vi "Servo Set Pulse Width N Channels.vi"(8 "Error In":errorcluster, 9 "Pulse Widths (uS)":u16[](array[numeric]), 10 "Servo Channels":u8[](array[numeric]), 11 "LINX Resource":T1) -> (0 "Error Out":errorcluster, 3 "LINX Resource":T1)   [LabVIEW 2014, in "LMH-LINX.lvlib" / "Servo.lvlib"]
doc: "Set the pulse width of the specified servo channel.\n\nA pulse width of 1500uS is typically the center point of rotation (90 degrees). Most servos can rotate between 1000 and 2000 uS but the actual limits will vary depending on the specific servo.s"
uses:
  <vilib>/MakerHub/LINX/Public/Sensors/Motion/Servo/Servo.lvlib
  <vilib>/MakerHub/LINX/Private/Type Defs/LINX Ref.ctl
  <vilib>/MakerHub/LINX/Private/Type Defs/Platform.ctl
  <vilib>/MakerHub/LINX/Private/Type Defs/Interface.ctl
  <vilib>/MakerHub/LINX/Private/Device/Type Defs/LINX Device Config.ctl
  <vilib>/MakerHub/LINX/Private/Device/Type Defs/TCP Config.ctl
  <vilib>/MakerHub/LINX/Private/Device/Type Defs/Channels.ctl
  <vilib>/MakerHub/LINX/Private/Type Defs/Peripheral.ctl
  <vilib>/MakerHub/LINX/Private/Type Defs/Error Type.ctl
  <vilib>/MakerHub/LINX/LMH-LINX.lvlib
  <vilib>/MakerHub/LINX/Private/Device/Device.lvlib
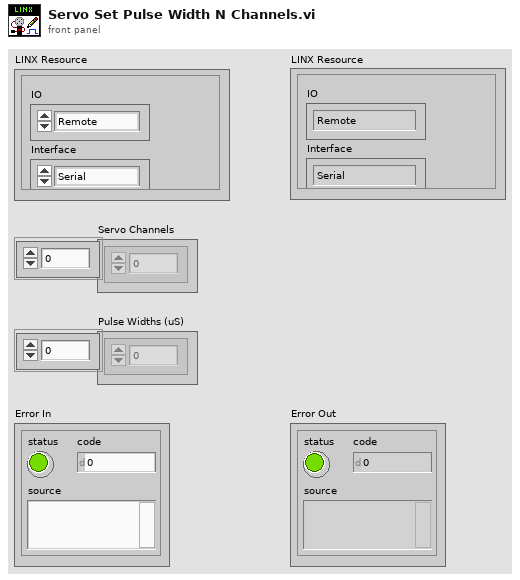
[diagram p1: front panel]
types:
  T1 = typedef "LMH-LINX.lvlib/LINX Ref.ctl" = cluster{"IO":T2, "Interface":T3, "LINX Device Config":T4}
  T2 = typedef "LMH-LINX.lvlib/Platform.ctl" = enum16{"Remote", "Local"}
  T3 = typedef "LMH-LINX.lvlib/Interface.ctl" = enum16{"Serial", "TCP"}
  T4 = typedef "LMH-LINX.lvlib/Device.lvlib/LINX Device Config.ctl" = cluster{"Interface":T3, "COM Port":refnum<visa-resource-name>, "TCP Configuration":T5, "Device Family":u8, "Device ID":u8, "Device Name":string, "TCP Ref":refnum<k5>, "Channels":T6}
  T5 = typedef "LMH-LINX.lvlib/Device.lvlib/TCP Config.ctl" = cluster{"IP Address":string, "Port":u16}
  T6 = typedef "LMH-LINX.lvlib/Channels.ctl" = cluster{"DI":u8[], "DO":u8[], "AI":u8[], "AO":u8[], "PWM":u8[], "QE":u8[], "UART":u8[], "I2C 2":u8[], "SPI":u8[], "CAN":u8[], "Servo":u8[], "AI Ref (V)":dbl, "AI Resolution (Bits)":u8, "AO Ref (V)":dbl, "AO Resolution (Bits)":u8}
  T7 = typedef "LMH-LINX.lvlib/Peripheral.ctl" = enum8{"DI", "DO", "AI", "AO", "PWM", "QE", "UART", "I2C", "SPI", "CAN", "Servo"}
  T8 = typedef "LMH-LINX.lvlib/Error Type.ctl" = enum16{"Unknown", "Timeout", "Corrupt Return Packet", "Unable To Connect", "Command Not Supported", "Channel DNE", "Invalid COM Config", "Firmware Version Mismatch", "myRIO Support", "CMD Specific Error", "Local IO Not Supported"}
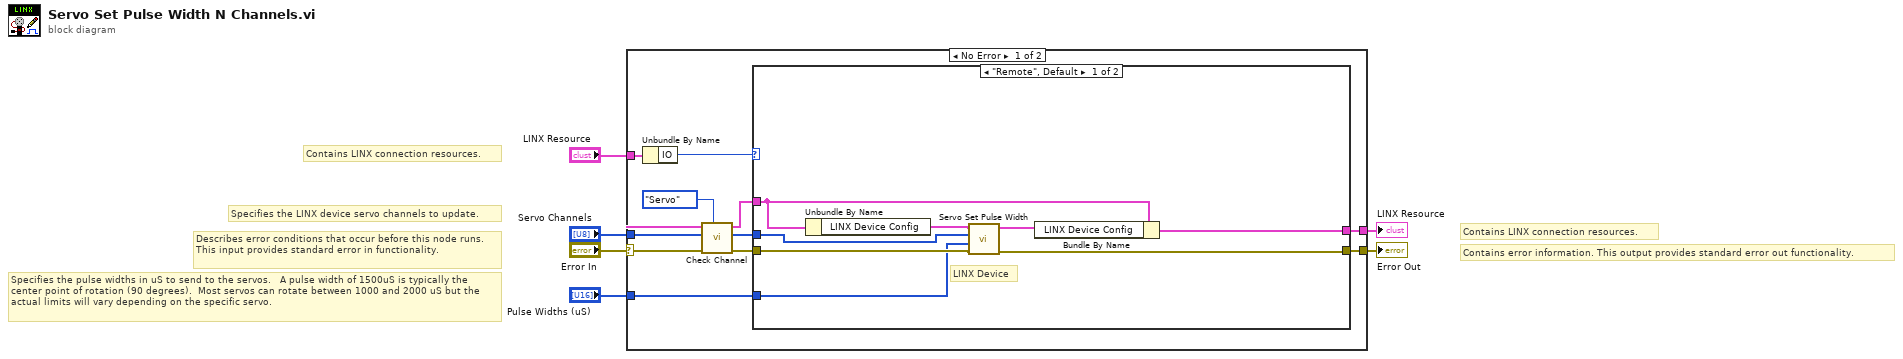
[diagram p0: block diagram]
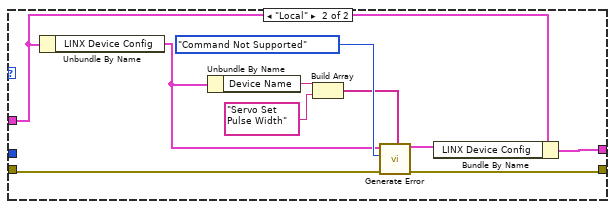
[diagram p2: hidden frame]
diagram:
  # "Specifies the pulse widths in uS to send to the servos.   A pulse width of 1500uS is typically the center point of rotation (90 degrees).  Most servos can rotate between 1000 and 2000 uS but the actual limits will vary depending on the specific servo."
  # "Specifies the LINX device servo channels to update."
  # "Contains LINX connection resources."
  # "Contains error information. This output provides standard error out functionality."
  # "Contains LINX connection resources."
  # "Describes error conditions that occur before this node runs. This input provides standard error in functionality."
  n1 = case shown="No Error" "Error In" {
    selector: "Error In" -> [w7 w37]
    tunnel: [w16 w37] -> w6
    tunnel: [w15 w36] -> w5
    tunnel: "LINX Resource" -> [w10 w36]
    tunnel: "Servo Channels" -> [w9 _]
    tunnel: "Pulse Widths (uS)" -> [w8 _]
    frame No Error {
      n2 = Unbundle By Name(w10) -> ("IO"=w17:T2)
      n3 = call <vilib>:"Check Channel.vi"("Peripheral"=Peripheral."Servo", "Error In"=w7, "Channels"=w9, "LINX Resource"=w10) -> ("Error Out"=w14:errorcluster, "Channels"=w13:u8[], "LINX Resource"=w11:T1)  [unwired: 5 in]
      n4 = case shown="\"Remote\", Default" w17 {
        tunnel: w14 -> [w21 w35]
        tunnel: w11 -> [w25 w28]
        tunnel: [w20 w34] -> w16
        tunnel: [w24 w26] -> w15
        tunnel: w13 -> [w19 _]
        tunnel: w8 -> [w18 _]
        frame "Remote", Default {
          # "LINX Device"
          n5 = Unbundle By Name(w25) -> ("LINX Device Config"=w23:T4)
          n6 = call <vilib>:"Servo Set Pulse Width.vi"("Error In"=w21, "Pulse Widths (uS)"=w18, "Channels"=w19, "LINX Device Config"=w23) -> ("Error Out"=w20:errorcluster, "LINX Device Config"=w22:T4)  [unwired: 6 in]
          n7 = Bundle By Name(cluster=w25, "LINX Device Config"=w22) -> (w24:T1)
        }
        frame "Local" {
          n8 = Unbundle By Name(w28) -> ("LINX Device Config"=w29:T4)
          n9 = Unbundle By Name(w29) -> ("Device Name"=w33:string)
          n10 = Build Array(w33, "Servo Set Pulse Width") -> (w30:string[])
          n11 = call <vilib>:"Generate Error.vi"("Error In"=w35, "Arguments"=w30, "Error Type"=Error_Type."Command Not Supported", "LINX Device Config"=w29) -> ("Error Out"=w34:errorcluster, "Dup LINX Device Config"=w27:T4)  [unwired: 6 in]
          n12 = Bundle By Name(cluster=w28, "LINX Device Config"=w27) -> (w26:T1)
        }
      }
    }
    frame Error {
    }
  }
  "Error Out" <- w6
  "LINX Resource" <- w5
